vi "Process Incoming Frames.vi"(6 "SignalValidRefs":T8, 7 "Incoming Session":refnum<k21>, 8 "error in":errorcluster, 9 "Incoming Signal Info":T1 {"Signal Settings Out"."Protection Configuration"."CRC Channels"."Data Type" items=["Signed", "Unsigned", "IEEE Float"]}, 10 "Incoming Signal Refs":T8, 11 "Incoming Frame Info In":T9) -> (0 "error out":errorcluster, 1 "Incoming Signal Info Out":T1 {"Signal Settings Out"."Protection Configuration"."CRC Channels"."Data Type" items=["Signed", "Unsigned", "IEEE Float"]}, 2 "Signal Values":dbl[](array[numeric]), 3 "Incoming Frame Info Out":T9, 5 "session out":refnum<k21>)   [LabVIEW 2015, in "Protection and Counter Addon Engine.lvlib"]
doc: "This example demonstrates receiving automatically converted values of signals, along with the associated timestamp value, using an NI-XNET Signal Input XY session. \n\nThis example can run against the CAN Signal Output XY example, assuming you have a properly terminated CAN cable connected to two CAN ports.\n\nIf you have no database aliases on your system, the example automatically loads the nixnet_example database."
uses:
  Protection and Counter Addon Engine.lvlib
  Users/Public/Documents/National Instruments/NI VeriStand 2015/Projects/Delete_Test_PaC_Incoming/LabVIEW/Incoming Frame Info.ctl
  <vilib>/NI/NIVS Inline Async API/_Data Access Engine/Data Access Engine/Types/Write.DVR.ctl
  <vilib>/NI/NIVS Inline Async API/_Data Access Engine/Access Type Classes/Write/Write.lvclass
  SubModules/Frame Protection Support/Source/Shared/Types/RT_Incoming_Signal_Info.ctl
  SubModules/Frame Protection Support/Source/Shared/Types/RT Exported Signal Settings.ctl
  SubModules/Frame Protection Support/Source/Shared/Types/Exported Counter Settings.ctl
  SubModules/Frame Protection Support/Source/Engine/Types/RT Protection Configuration.ctl
  SubModules/Frame Protection Support/Source/Shared/Types/Protection Type.ctl
  SubModules/Frame Protection Support/Source/Shared/Types/XNET Signal Configuration.ctl
  <vilib>/NI/NIVS Inline Async API/_Data Access Engine/Access Type Classes/Write/Write.lvclass/Write.ctl
  <vilib>/NI/NIVS Inline Async API/_Data Access Engine/Data Access Engine/Methods/Write.Data.vi
  <vilib>/NI/NIVS Inline Async API/_Data Access Engine/Access Type Classes/Write/Write.ProcessData.vi
  <vilib>/xnet/xnet.llb/XNET Read (Signal XY).vi
  <vilib>/NI/NIVS Inline Async API/_Data Access Engine/Data Access Engine/Data Access Engine.lvclass
  SubModules/Frame Protection Support/Source/Shared/Protection and Counter Support Shared.lvlib
  SubModules/Frame Protection Support/Source/Engine/Protection and Counter Support Engine.lvlib
panel:
  out "counter valid":bool
  out "data 2":T7(array[cluster])
  out "Delta t":dbl
  out "Frame Receive Time":timestamp
  out "data":T7(array[cluster])
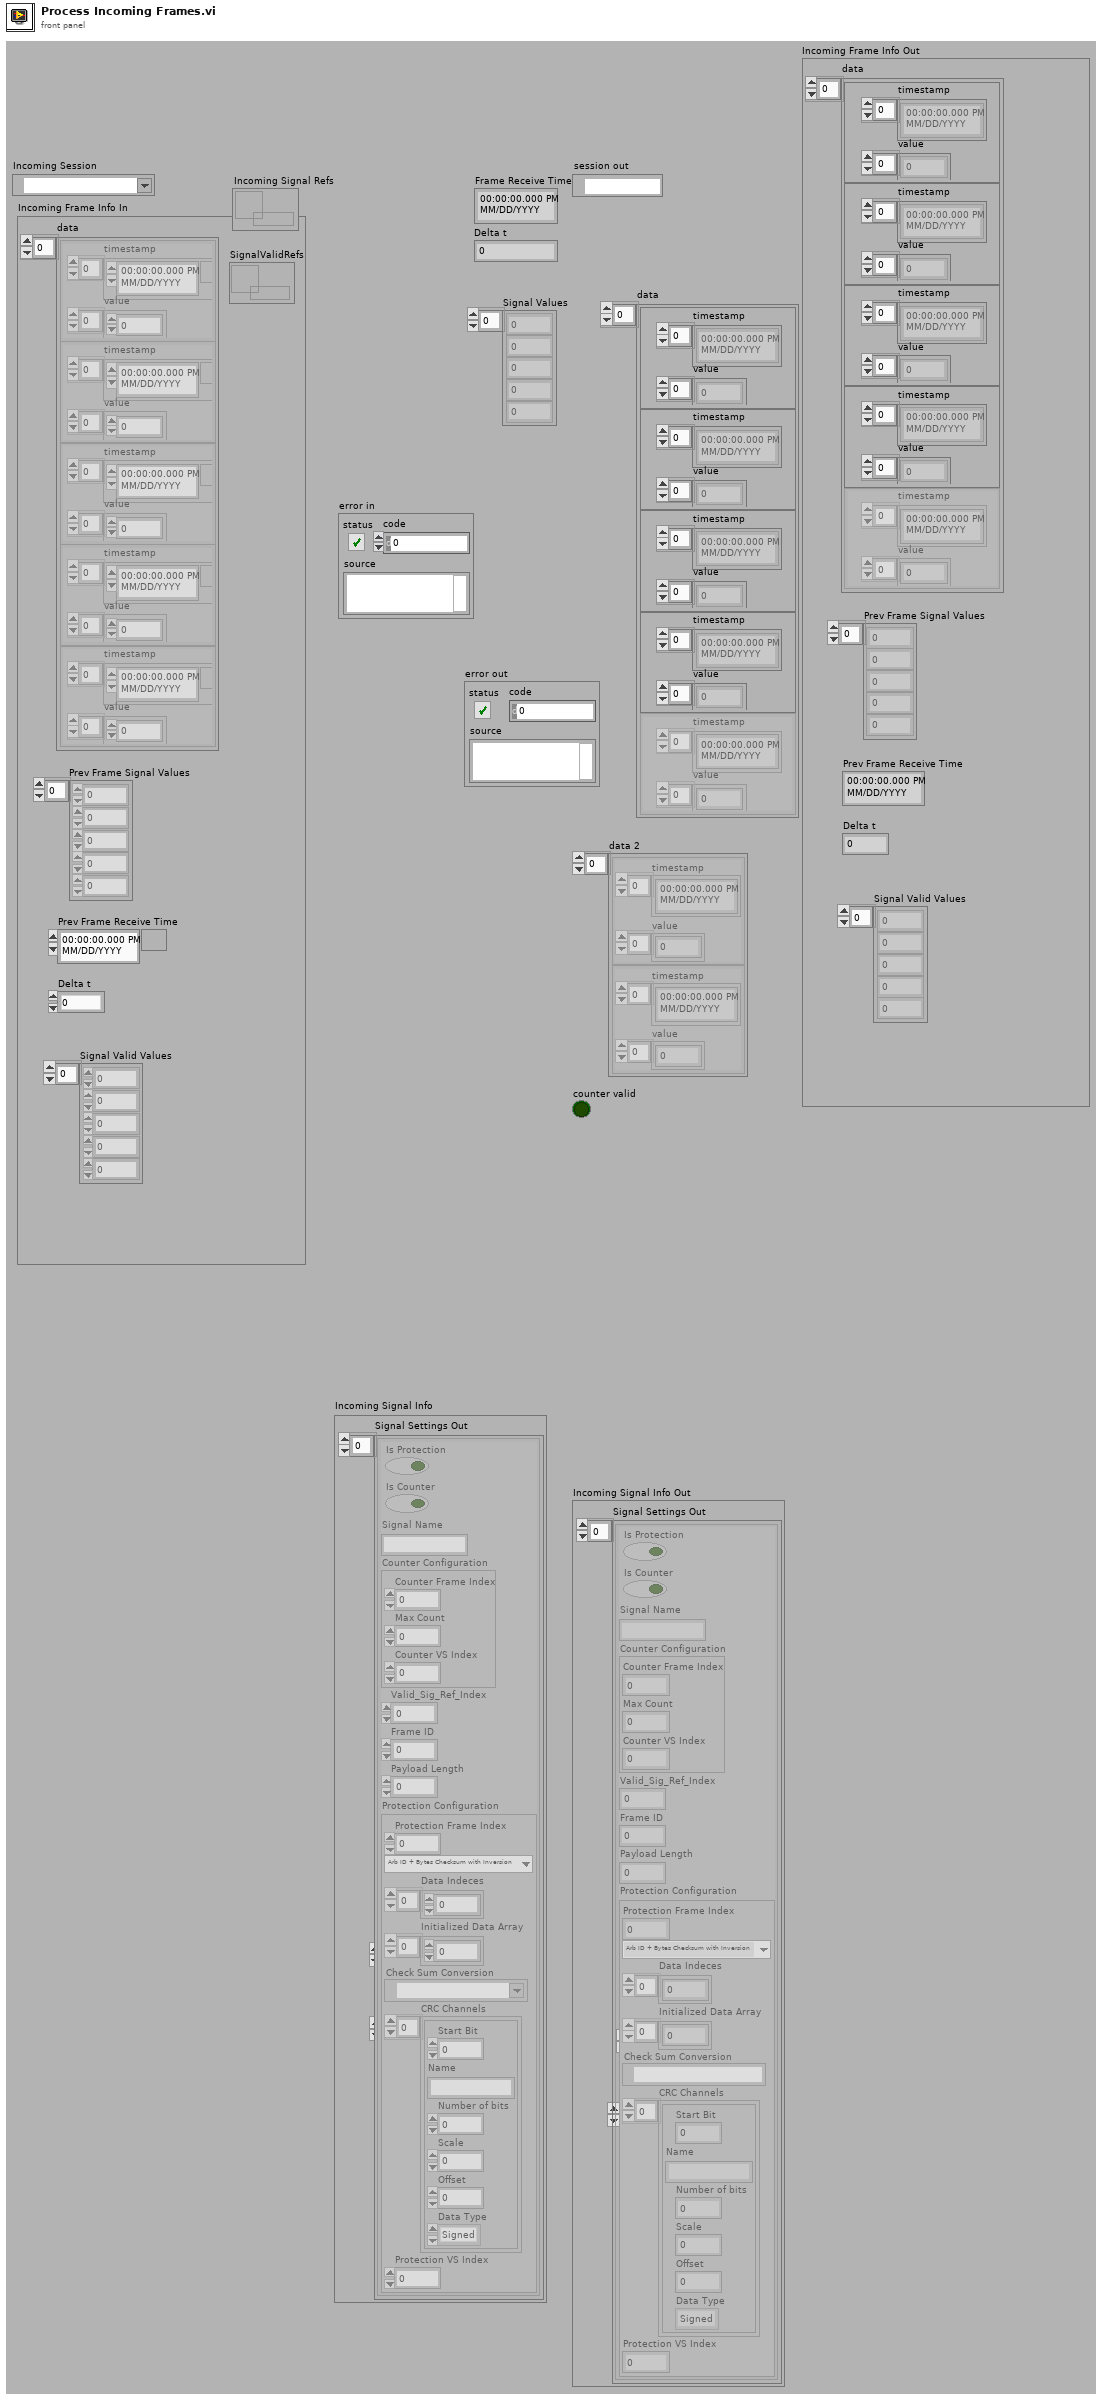
[diagram p1: front panel]
types:
  T1 = typedef "Protection and Counter Support Shared.lvlib/RT_Incoming_Signal_Info.ctl" = cluster{"Signal.PrevData":dbl[], "Signal Names":string[], "Signal Settings Out":T2[]}
  T2 = typedef "Protection and Counter Support Shared.lvlib/RT Exported Signal Settings.ctl" = cluster{"Is Protection":bool, "Is Counter":bool, "Signal Name":string, "Counter Configuration":T3, "Valid_Sig_Ref_Index":i32, "Frame ID":u32, "Payload Length":u32, "Protection Configuration":T4}
  T3 = typedef "Protection and Counter Support Shared.lvlib/Exported Counter Settings.ctl" = cluster{"Counter Frame Index":i32, "Max Count":dbl, "Counter VS Index":i32}
  T4 = typedef "Protection and Counter Support Engine.lvlib/RT Protection Configuration.ctl" = cluster{"Protection Frame Index":i32, "Protection Type":T5, "Data Indeces":i32[], "Initialized Data Array":dbl[], "Check Sum Conversion":refnum<k21>, "CRC Channels":T6[], "Protection VS Index":i32}
  T5 = typedef "Protection and Counter Support Shared.lvlib/Protection Type.ctl" = enum16{"Arb ID + Bytes Checksum with Inversion", "Arb ID + Bytes CRC with Inversion", "Reversed Raw Signal Checksum with Inversion"}
  T6 = typedef "Protection and Counter Support Shared.lvlib/XNET Signal Configuration.ctl" = cluster{"Start Bit":i32, "Name":string, "Number of bits":i32, "Scale":dbl, "Offset":dbl, "Data Type":u32}
  T7 = cluster{"timestamp":timestamp[], "value":dbl[]}[]
  T8 = typedef "Data Access Engine.lvlib/Data Access Engine.lvclass/Write.DVR.ctl" = refnum<data-value>
  T9 = typedef "Protection and Counter Addon Engine.lvlib/Incoming Frame Info.ctl" = cluster{"data":cluster{"timestamp":timestamp[], "value":dbl[]}[], "Prev Frame Signal Values":dbl[], "Prev Frame Receive Time":timestamp, "Delta t":dbl, "Signal Valid Values":dbl[]}
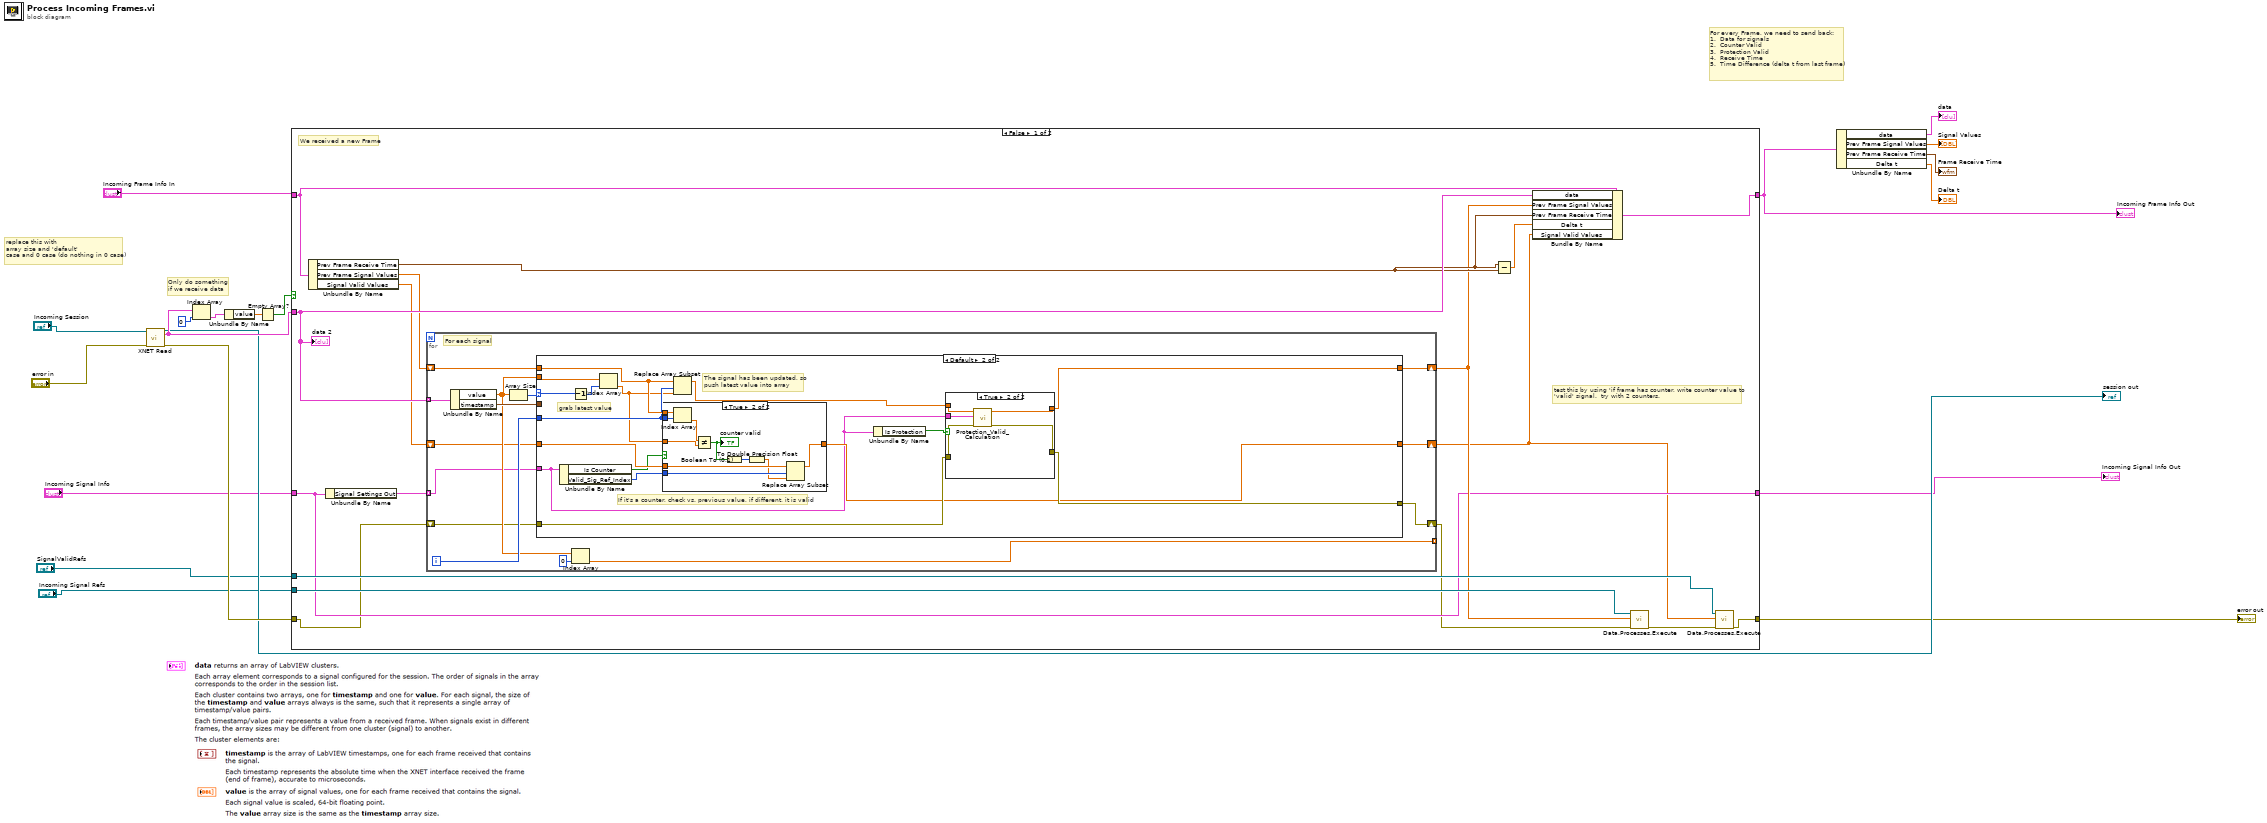
[diagram p0: block diagram]
diagram:
  # "replace this with\narray size and 'default'\ncase and 0 case (do nothing in 0 case)"
  # "Only do something\nif we receive data"
  # "For every Frame, we need to send back:\n1.  Data for signals\n2.  Counter Valid\n3.  Protection Valid\n4.  Receive Time\n5.  Time Difference (delta t from last frame)"
  n1 = call-poly <vilib>:"XNET Read.vi"("session in"="Incoming Session", "error in (no error)"="error in") -> ("session out"=→"session out":refnum<k21>, "data"=w15:T7, "error out"=w16:errorcluster)  [unwired: 11 out]
  n2 = Index Array(array=w15, index=0) -> (element=w13:cluster{"timestamp":timestamp[], "value":dbl[]})
  n3 = Unbundle By Name(w13) -> ("value"=w12:dbl[])
  n4 = Empty Array?(array=w12) -> (empty?=w11:bool)
  n5 = case shown="False" w11 {
    tunnel: w15 -> [w37 _]
    tunnel: w16 -> [w22 w91]
    tunnel: [w33 w91] -> w5
    tunnel: "Incoming Frame Info In" -> [w30 w90]
    tunnel: [w36 w90] -> w17
    tunnel: "Incoming Signal Refs" -> [w32 _]
    tunnel: "SignalValidRefs" -> [w31 _]
    tunnel: "Incoming Signal Info" -> [w26 w89]
    tunnel: [w26 w89] -> w1
    frame False {
      # "test this by using 'if frame has counter, write counter value to\n'valid' signal.  try with 2 counters."
      # "We received a new Frame"
      n6 = Unbundle By Name(w30) -> ("Prev Frame Receive Time"=w29:timestamp, "Prev Frame Signal Values"=w27:dbl[], "Signal Valid Values"=w24:dbl[])
      n7 = Unbundle By Name(w26) -> ("Signal Settings Out"=w25:T2[])
      n8 = for {
        tunnel: w37 -> [w51] mode=indexing
        shift-right: [w47] -> w28
        shift-left: w27 -> [w48]
        tunnel: [w43] -> _ mode=indexing
        tunnel: w25 -> [w42] mode=indexing
        shift-right: [w40] -> w23
        shift-left: w24 -> [w41]
        shift-right: [w38] -> w21
        shift-left: w22 -> [w39]
        i -> [w46]
        # "For each signal"
        n9 = Unbundle By Name(w51) -> ("value"=w45:dbl[], "timestamp"=w49:timestamp[])
        n10 = Array Size(array=w45) -> (size(s)=w50:i32)
        n11 = case shown="Default" w50 {
          selector: w50 -> [_ w70]
          tunnel: w49 -> [_ _]
          tunnel: w48 -> [w54 w67]
          tunnel: [w54 w57] -> w47
          tunnel: w45 -> [_ w69]
          tunnel: w46 -> [_ w66]
          tunnel: w42 -> [_ w56]
          tunnel: w41 -> [w53 w64]
          tunnel: [w53 w59] -> w40
          tunnel: w39 -> [w52 w61]
          tunnel: [w52 w60] -> w38
          frame 0 {
            # "The signal has not been updated, so\npass through previous value"
          }
          frame Default {
            # "If it's a counter, check vs. previous value, if different, it is valid"
            # "The signal has been updated, so\npush latest value into array"
            # "grab latest value"
            n12 = Unbundle By Name(w56) -> ("Is Counter"=w62:bool, "Valid_Sig_Ref_Index"=w63:i32)
            n13 = Decrement(x=w70) -> (x-1=w68:i32)
            n14 = Index Array(array=w69, index=w68) -> (element=w65:dbl)
            n15 = case shown="True" w62 {
              tunnel: w67 -> [_ w88]
              tunnel: w66 -> [_ w87]
              tunnel: w65 -> [_ w85]
              tunnel: w64 -> [w78 w82]
              tunnel: w63 -> [_ w81]
              tunnel: [w78 w79] -> w59
              frame False {
              }
              frame True {
                n16 = Index Array(array=w88, index=w87) -> (element=w86:dbl)
                n17 = Not Equal?(x=w86, y=w85) -> (x != y?=w84:bool)
                "counter valid" <- w84
                n18 = Boolean To (0,1)(Boolean=w84) -> (0, 1=w83:i16)
                n19 = To Double Precision Float(number=w83) -> (double precision float=w80:dbl)
                n20 = Replace Array Subset(array=w82, new element=w80, index=w81) -> (w79:dbl[])
              }
            }
            n21 = Replace Array Subset(array=w67, new element=w65, index=w66) -> (w58:dbl[])
            n22 = Unbundle By Name(w56) -> ("Is Protection"=w55:bool)
            n23 = case shown="True" w55 {
              tunnel: w61 -> [w71 w77]
              tunnel: [w71 w76] -> w60
              tunnel: w58 -> [w72 w75]
              tunnel: [w72 w74] -> w57
              tunnel: w56 -> [_ w73]
              frame False {
              }
              frame True {
                n24 = call "Protection_Valid_Calculation.vi"("error in"=w77, "Signal Settings"=w73, "Signal Values In"=w75) -> ("error out"=w76:errorcluster, "Signal Values Out"=w74:dbl[])  [unwired: 7 in]
              }
            }
          }
        }
        n25 = Index Array(array=w45, index=0) -> (element=w43:dbl)
      }
      n26 = Subtract(x=w29, y=w29) -> (x-y=w35:dbl)
      n27 = Bundle By Name(cluster=w30, "data"=w37, "Prev Frame Signal Values"=w28, "Prev Frame Receive Time"=w29, "Delta t"=w35, "Signal Valid Values"=w23) -> (w36:T9)
      n28 = call-poly <vilib>:"Data.Processes.Execute.vi"("error in (no error)"=w21, "Values"=w28, "Ref"=w32) -> ("error out"=w34:errorcluster)  [unwired: 8 in]
      n29 = call-poly <vilib>:"Data.Processes.Execute.vi"("error in (no error)"=w34, "Values"=w23, "Ref"=w31) -> ("error out"=w33:errorcluster)  [unwired: 8 in]
      "data 2" <- w37
    }
    frame True {
      # "No Frame Received"
    }
  }
  "Incoming Frame Info Out" <- w17
  "error out" <- w5
  "Incoming Signal Info Out" <- w1
  n30 = Unbundle By Name(w17) -> ("data"=→"data":T7, "Prev Frame Signal Values"=→"Signal Values":dbl[], "Prev Frame Receive Time"=→"Frame Receive Time":timestamp, "Delta t"=→"Delta t":dbl)
